vi "Create Pulse Output.vi"(8 "error in (no error)":errorcluster, 10 "Params":variant, 11 "NI Counter Output in":refnum<class "NI Counter Output.lvclass">) -> (0 "error out":errorcluster, 3 "NI Counter Output out":refnum<class "NI Counter Output.lvclass">)   [LabVIEW 2020, in "NI DAQmx.lvlib" / "NI Counter Output.lvclass"]
uses:
  NI Counter Output.lvclass
  D:/WSGitHub/RTFWK/Realization/NI DAQmx Base/NI DAQmx Base.lvclass
  TypeDefs/Pulse output.ctl
  <vilib>/DAQmx/create/channels.llb/DAQmx Create Channel (CO-Pulse Generation-Frequency).vi
  <vilib>/DAQmx/configure/timing.llb/DAQmx Timing (Implicit).vi
  NI Counter Output.lvclass/NI Counter Output.ctl
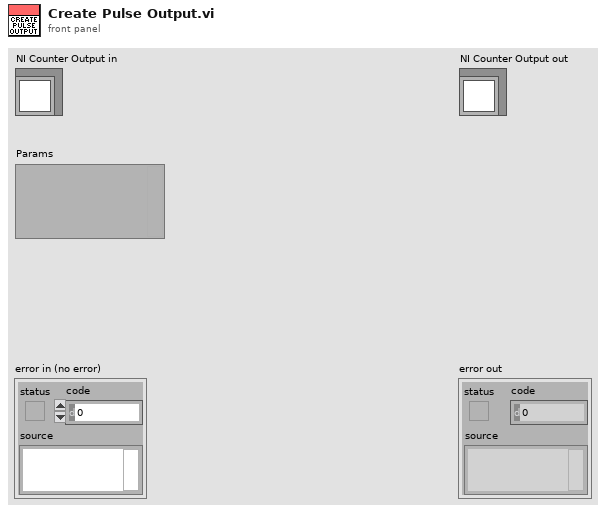
[diagram p1: front panel]
types:
  T1 = typedef "Pulse output.ctl" = cluster{"channel":string, "duty cycle":dbl, "frequency":dbl, "pulses":i32, "initial delay":dbl}
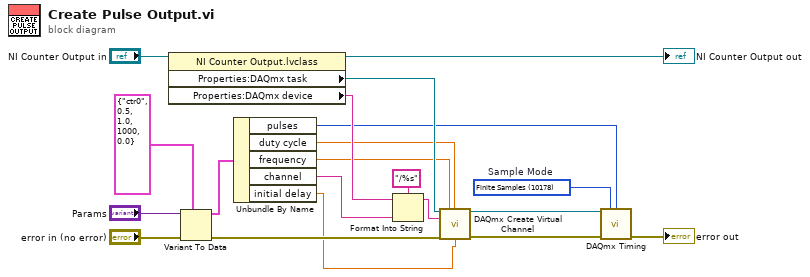
[diagram p0: block diagram]
diagram:
  w16 = 10178 items=["Finite Samples"=10178, "Continuous Samples"=10123, "Hardware Timed Single Point"=12522]  # Sample Mode
  n1 = property class="NI Counter Output.lvclass"(reference="NI Counter Output in") -> (reference out=→"NI Counter Output out":refnum<class "NI Counter Output.lvclass">, "Properties:DAQmx task"=w12:refnum<k21>, "Properties:DAQmx device"=w7:tag)  [unwired: 1 in, 1 out]
  n2 = Variant To Data(error in="error in (no error)", type=T1 {"channel"="ctr0", "duty cycle"=0.5, "frequency"=1.0, "pulses"=1000, "initial delay"=0.0}, Variant="Params") -> (data=w6:T1, error out=w10:errorcluster)
  n3 = Unbundle By Name(w6) -> ("pulses"=w1:i32, "duty cycle"=w3:dbl, "frequency"=w2:dbl, "channel"=w5:string, "initial delay"=w4:dbl)
  n4 = Format Into String(format string="/%s", initial string=w7, w5) -> (resulting string=w8:string)  [unwired: 1 in, 1 out]
  n5 = call-poly <vilib>:"DAQmx Create Virtual Channel.vi"("task in"=w12, "frequency"=w2, "duty cycle"=w3, "counter"=w8, "error in"=w10, "initial delay"=w4) -> ("task out"=w15:refnum<k21>, "error out"=w14:errorcluster)  [unwired: 8 in]
  n6 = call-poly <vilib>:"DAQmx Timing.vi"("task/channels in"=w15, "sample mode"=w16, "samples per channel"=w1, "error in"=w14) -> ("error out"=→"error out":errorcluster)  [unwired: 10 in, 1 out]
